vi "Winch Controller.vi"(8 "error in":errorcluster) -> ()   [LabVIEW 2016]
doc: "This VI executes continuously carrying out the current operation and responding to updates or new operations. It will often contain the timing or control code that is difficult to place directly in TeleOp. This VI generally opens all sensors and motors and isolates the rest of the robot code from knowing how the operations are carried out."
uses:
  Winch Setpoints.ctl
  Winch Operations.ctl
  <vilib>/Rock Robotics/SystemInterfaces/DIO/FPGA_DIOPWMChannel.ctl
  <vilib>/Rock Robotics/WPI/MotorControl/WPI_MotorControlOpen Victor.vi
  <vilib>/Rock Robotics/Network Tables/NT Write Boolean.vi
panel:
  out "Current\nCmd":string
  # "Tip: It may be helpful to observe inputs and sensor values.\nYou may also want to display tuning or debugging controls."
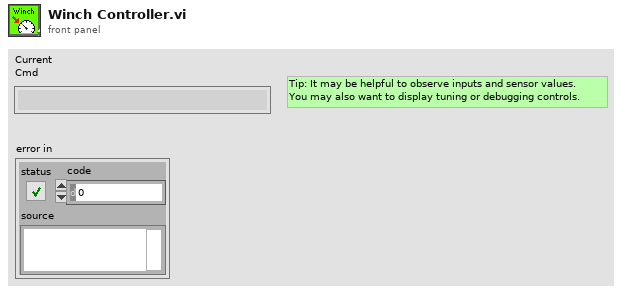
[diagram p1: front panel]
types:
  T1 = typedef "FPGA_DIOPWMChannel.ctl" = enum8{"PWM 0", "PWM 1", "PWM 2", "PWM 3", "PWM 4", "PWM 5", "PWM 6", "PWM 7", "PWM 8", "PWM 9", "PWM MXP 0", "PWM MXP 1", "PWM MXP 2", "PWM MXP 3", "PWM MXP 4", "PWM MXP 5", "PWM MXP 6", "PWM MXP 7", "PWM MXP 8", "PWM MXP 9", "Invalid"}
  T2 = typedef "Winch Setpoints.ctl" = cluster{"Operation":T3, "Speed":dbl}
  T3 = typedef "Winch Operations.ctl" = enum16{"Reserve", "Read Current", "Immediate", "Go up, Go down"}
  T4 = typedef "Command Status Info.ctl" = cluster{"Name":string, "Status":T5, "notifier out":T6}
  T5 = typedef "Completion Status.ctl" = enum16{"Successful", "Aborted", "Incomplete"}
  T6 = typedef "Completion Notifier.ctl" = refnum<notifier>
  T7 = cluster{"Default Command":T2, "Command Timing":cluster{"Start Time (ms)":u32, "Iterations":i32}, "Command Arguments":cluster{"Command Info":T4, "Description":string, "Default Command":T2, "notifier out":refnum<notifier>, "Subsystem Name":string}}
  T8 = typedef "WPI_MotorControlDeviceRef.ctl" = cluster{"DeviceStatus":errorcluster, "Type":T9, "PWM":cluster{"PWM Channel":T1, "DeadBand":T10}, "CAN":cluster{"Device Number":u8, "SetOutput VI Ref":variant, "GetOutput VI Ref":variant, "Enable VI Ref":variant, "Disable VI Ref":variant, "Data":variant}, "Invert":bool}
  T9 = typedef "WPI_MotorControlType.ctl" = enum16{"PWM", "CAN"}
  T10 = typedef "WPI_PWMDeadband.ctl" = cluster{"Name":string, "maxPositivePwm":i32, "minPositivePwm":i32, "centerPwm":i32, "maxNegativePwm":i32, "minNegativePwm":i32, "angularRange":u16}
  T11 = cluster{"Device Number":u8, "SetOutput VI Ref":variant, "GetOutput VI Ref":variant, "Enable VI Ref":variant, "Disable VI Ref":variant, "Data":variant}
  T12 = cluster{"DeviceStatus":errorcluster, "Type":T9, "PWM":cluster{"PWM Channel":T1, "DeadBand":T10}, "CAN":cluster{"Device Number":u8, "SetOutput VI Ref":variant, "GetOutput VI Ref":variant, "Enable VI Ref":variant, "Disable VI Ref":variant, "Data":variant}, "Invert":bool}
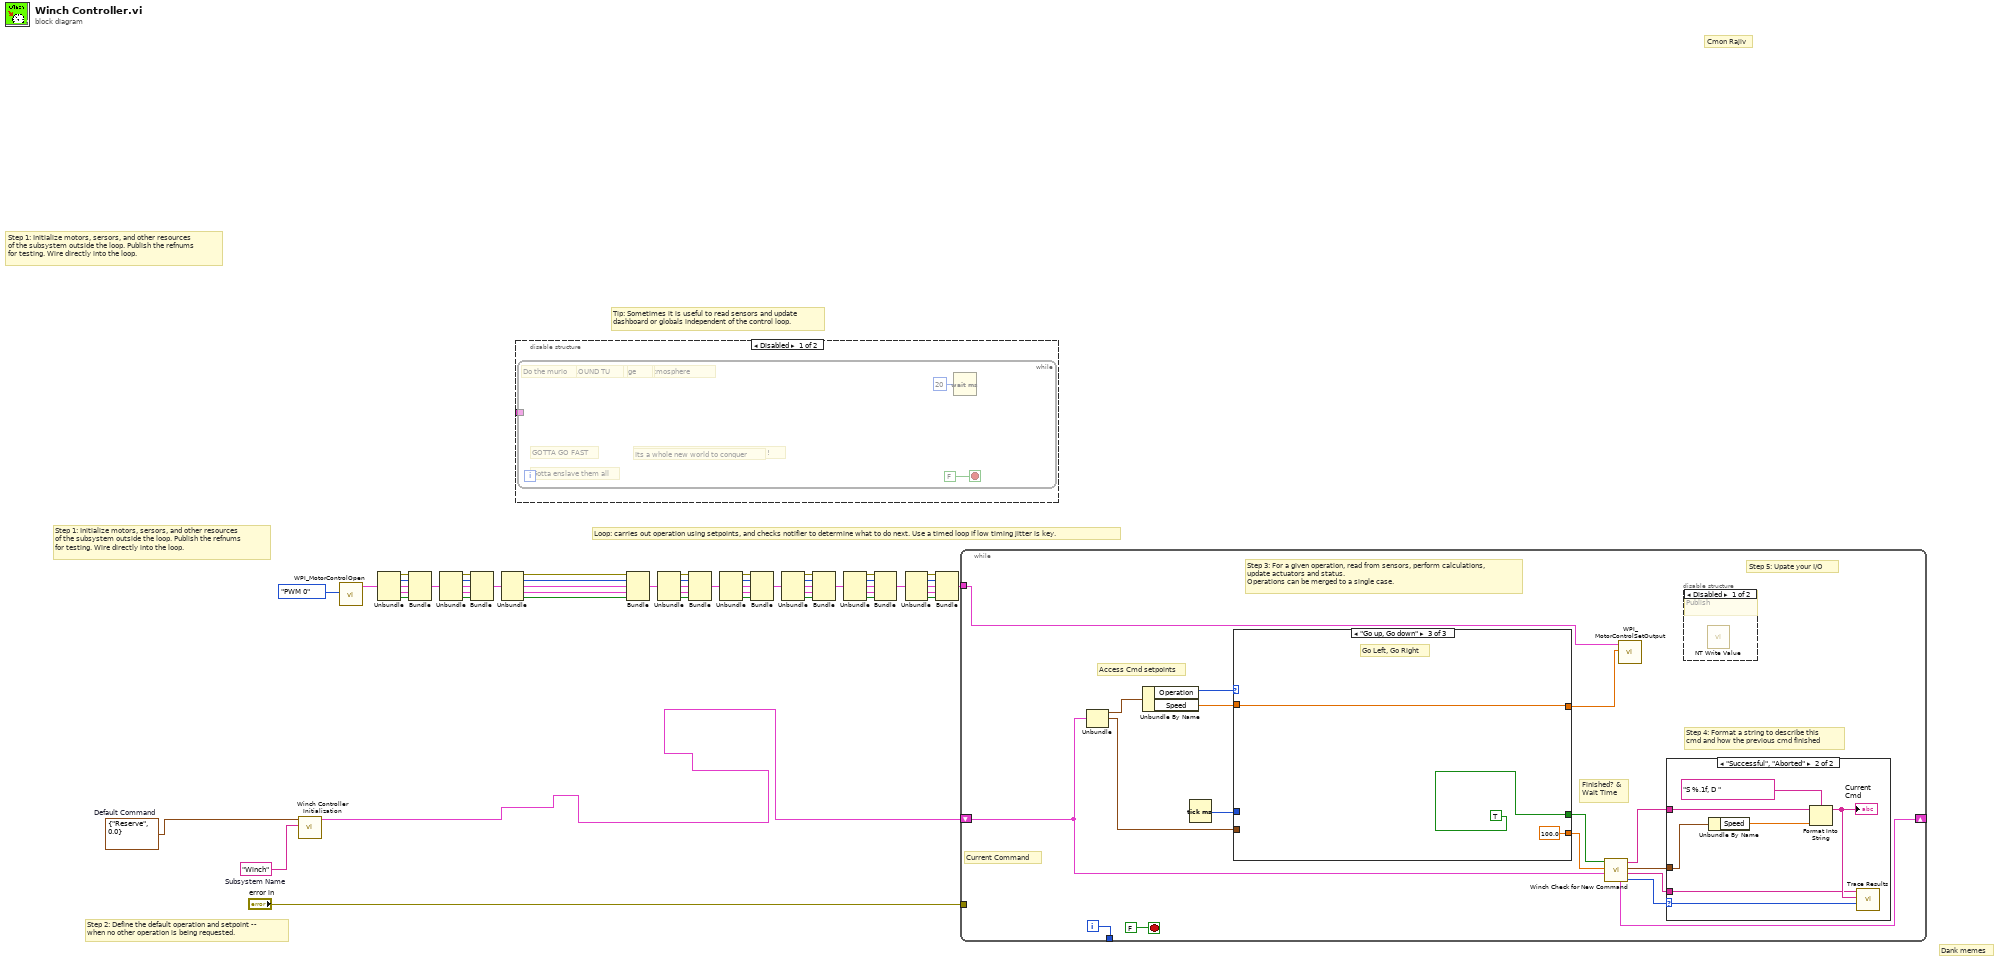
[diagram p0: block diagram]
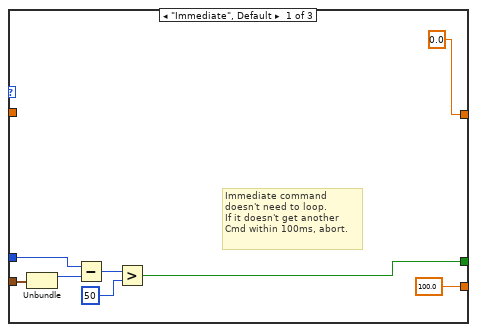
[diagram p5: hidden frame]
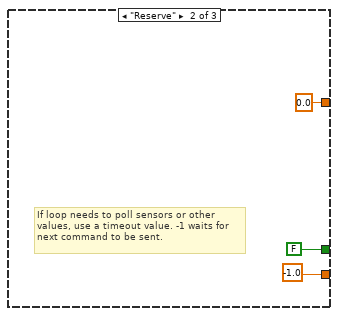
[diagram p6: hidden frame]
diagram:
  w2 = T2 {"Operation"=enum."Reserve", "Speed"=0.0}  # Default Command
  w53 = "Winch"  # Subsystem Name
  # "Step 1: Initialize motors, sersors, and other resources\nof the subsystem outside the loop. Publish the refnums\nfor testing. Wire directly into the loop."
  # "Cmon Rajiv"
  # "Dank memes"
  # "Tip: Sometimes it is useful to read sensors and update\ndashboard or globals independent of the control loop."
  # "Step 2: Define the default operation and setpoint --\nwhen no other operation is being requested."
  # "Step 1: Initialize motors, sersors, and other resources\nof the subsystem outside the loop. Publish the refnums\nfor testing. Wire directly into the loop."
  # "Loop: carries out operation using setpoints, and checks notifier to determine what to do next. Use a timed loop if low timing jitter is key."
  n1 = call "Winch Controller Initialization.vi"("Subsystem Name"=w53, "Default Command"=w2) -> ("Command Info"=w1:T7)  [unwired: 9 in]
  n2 = call-poly <vilib>:"WPI_MotorControlOpen.vi"("PWM Channel"=FPGA_DIOPWMChannel."PWM 0") -> ("MotorControlDeviceRef"=w51:T8)  [unwired: 9 in, 1 out]
  n3 = Unbundle(w51) -> ("DeviceStatus"=w50:errorcluster, "Type"=w49:T9, "PWM"=w48:cluster{"PWM Channel":T1, "DeadBand":T10}, "CAN"=w47:T11, "Invert"=w46:bool)
  n4 = Bundle("DeviceStatus"=w50, "Type"=w49, "PWM"=w48, "CAN"=w47, "Invert"=w46) -> (w40:T12)  [unwired: 1 in]
  n5 = Unbundle(w40) -> ("DeviceStatus"=w45:errorcluster, "Type"=w44:T9, "PWM"=w43:cluster{"PWM Channel":T1, "DeadBand":T10}, "CAN"=w42:T11, "Invert"=w41:bool)
  n6 = Bundle("DeviceStatus"=w45, "Type"=w44, "PWM"=w43, "CAN"=w42, "Invert"=w41) -> (w28:T12)  [unwired: 1 in]
  n7 = Unbundle(w28) -> ("DeviceStatus"=w39:errorcluster, "Type"=w38:T9, "PWM"=w37:cluster{"PWM Channel":T1, "DeadBand":T10}, "CAN"=w36:T11, "Invert"=w35:bool)
  n8 = disable-structure shown="Disabled" {
    disable-tunnel: _ -> [w55 _]
    frame Disabled {
      n9 = while {
        tunnel: w55 -> [_]
        stop <- FALSE stop-if-true
        # "Who lives in a watermelon under the atmosphere"
        # "Its a whole new world to conquer"
        # "It's not always yellow and orange"
        # "Do you wana be a master of slavery??!!"
        # "We all live, in a Smokemon World"
        # "Gotta enslave them all"
        # "GOTTA GO FAST"
        # "KURBU LEFT AROUND TU"
        # "SANIC UNDERGROUUUND"
        # "Do the murio"
        n10 = Wait (ms)(milliseconds to wait=u32 20) -> ()  [unwired: 1 out]
      }
    }
    frame Enabled {
    }
  }
  n11 = Bundle("DeviceStatus"=w39, "Type"=w38, "PWM"=w37, "CAN"=w36, "Invert"=w35) -> (w29:T12)  [unwired: 1 in]
  n12 = Unbundle(w29) -> ("DeviceStatus"=w34:errorcluster, "Type"=w33:T9, "PWM"=w32:cluster{"PWM Channel":T1, "DeadBand":T10}, "CAN"=w31:T11, "Invert"=w30:bool)
  n13 = Bundle("DeviceStatus"=w34, "Type"=w33, "PWM"=w32, "CAN"=w31, "Invert"=w30) -> (w4:T12)  [unwired: 1 in]
  n14 = Unbundle(w4) -> ("DeviceStatus"=w16:errorcluster, "Type"=w15:T9, "PWM"=w14:cluster{"PWM Channel":T1, "DeadBand":T10}, "CAN"=w13:T11, "Invert"=w12:bool)
  n15 = Bundle("DeviceStatus"=w16, "Type"=w15, "PWM"=w14, "CAN"=w13, "Invert"=w12) -> (w6:T12)  [unwired: 1 in]
  n16 = Unbundle(w6) -> ("DeviceStatus"=w11:errorcluster, "Type"=w10:T9, "PWM"=w9:cluster{"PWM Channel":T1, "DeadBand":T10}, "CAN"=w8:T11, "Invert"=w7:bool)
  n17 = Bundle("DeviceStatus"=w11, "Type"=w10, "PWM"=w9, "CAN"=w8, "Invert"=w7) -> (w5:T12)  [unwired: 1 in]
  n18 = Unbundle(w5) -> ("DeviceStatus"=w27:errorcluster, "Type"=w26:T9, "PWM"=w25:cluster{"PWM Channel":T1, "DeadBand":T10}, "CAN"=w24:T11, "Invert"=w23:bool)
  n19 = Bundle("DeviceStatus"=w27, "Type"=w26, "PWM"=w25, "CAN"=w24, "Invert"=w23) -> (w17:T12)  [unwired: 1 in]
  n20 = Unbundle(w17) -> ("DeviceStatus"=w22:errorcluster, "Type"=w21:T9, "PWM"=w20:cluster{"PWM Channel":T1, "DeadBand":T10}, "CAN"=w19:T11, "Invert"=w18:bool)
  n21 = Bundle("DeviceStatus"=w22, "Type"=w21, "PWM"=w20, "CAN"=w19, "Invert"=w18) -> (w3:T12)  [unwired: 1 in]
  n22 = while {
    shift-right: [w67] -> _
    shift-left: w1 -> [w68]
    tunnel: [w73] -> _
    tunnel: "error in" -> [_]
    tunnel: w3 -> [w58]
    i -> [w73]
    stop <- FALSE stop-if-true
    # "Step 5: Upate your I/O"
    # "Step 4: Format a string to describe this\ncmd and how the previous cmd finished"
    # "Current Command"
    # "Access Cmd setpoints"
    # "Finished? &\nWait Time"
    # "Step 3: For a given operation, read from sensors, perform calculations,\nupdate actuators and status.\nOperations can be merged to a single case."
    n23 = Unbundle(w68) -> ("Default Command"=w72:T2, "Command Timing"=w69:cluster{"Start Time (ms)":u32, "Iterations":i32})  [unwired: 1 out]
    n24 = Unbundle By Name(w72) -> ("Operation"=w71:T3, "Speed"=w60:dbl)
    n25 = Tick Count (ms)() -> (millisecond timer value=w70:u32)
    n26 = case shown="\"Go up, Go down\"" w71 {
      tunnel: [100.0 -1.0 100.0] -> w65
      tunnel: [w83 FALSE ("ignore previous (F)") TRUE ("ignore previous (F)")] -> w66
      tunnel: w69 -> [w85 _ _]
      tunnel: w70 -> [w84 _ _]
      tunnel: w60 -> [_ _ w95]
      tunnel: [0.0 0.0 w95] -> w59
      frame "Immediate", Default {
        # "Immediate command\ndoesn't need to loop.\nIf it doesn't get another\nCmd within 100ms, abort."
        n27 = Unbundle(w85) -> ("Start Time (ms)"=w88:u32)  [unwired: 1 out]
        n28 = Subtract(x=w84, y=w88) -> (x-y=w87:u32)
        n29 = Greater?(x=w87, y=u8 50 ("Left Motor")) -> (0:w83:bool)
      }
      frame "Reserve" {
        # "If loop needs to poll sensors or other\nvalues, use a timeout value. -1 waits for\nnext command to be sent."
      }
      frame "Go up, Go down" {
        # "Go Left, Go Right"
      }
    }
    n30 = call "Winch Check for New Command.vi"("Current Command"=w68, "Wait time (ms)"=w65, "Finished?"=w66) -> ("Completion"=w61:T5, "Subsystem Name"=w62:string, "Current Command"=w63:T2, "Initial Trace String"=w64:string, "NextCommand"=w67:T7)  [unwired: 4 in]
    n31 = call <vilib>:"WPI_MotorControlSetOutput.vi"("Output"=w59, "MotorControlDevRef"=w58) -> ()  [unwired: 7 in, 3 out]
    n32 = case shown="\"Successful\", \"Aborted\"" w61 {
      selector: w61 -> [_ w81]
      tunnel: w64 -> [_ w77]
      tunnel: w63 -> [_ w78]
      tunnel: w62 -> [_ w75]
      frame "Incomplete", Default {
        # "Continuing current command"
      }
      frame "Successful", "Aborted" {
        # "Report and setup for next command"
        n33 = Unbundle By Name(w78) -> ("Speed"=w80:dbl)
        n34 = Format Into String(format string="S %.1f, D ", initial string=w77, w80) -> (resulting string=w76:string)  [unwired: 1 in, 1 out]
        "Current\nCmd" <- w76
        n35 = call <vilib>:"Trace Results.vi"("Status of previous command"=w81, "Description"=w76, "Subsystem"=w75) -> ()  [unwired: 9 in]
      }
    }
    n36 = disable-structure shown="Disabled" {
      frame Disabled {
        # "Publish"
        n37 = call-poly <vilib>:"NT Write Value.vi"() -> ()  [unwired: 11 in, 1 out]
      }
      frame Enabled {
      }
    }
  }
